vi "Read.vi"(7 "I2C Channel (0)":u8, 8 "Error In":errorcluster, 10 "TCN75A I2C Address":T7, 11 "LINX Resource":T1) -> (0 "Error Out":errorcluster, 1 "Temp F":dbl, 2 "Temp C":dbl, 3 "LINX Resource":T1)   [LabVIEW 2011, in "LVH-LINX.lvlib" / "TCN75A.lvlib"]
doc: "Read temperature from the TCN75A."
uses:
  TCN75A.lvlib
  Private/Type Defs/LINX Ref.ctl
  Private/Type Defs/Platform.ctl
  Private/Type Defs/Interface.ctl
  Private/Device/Type Defs/LINX Device Config.ctl
  Private/Device/Type Defs/TCP Config.ctl
  Private/Device/Type Defs/Channels.ctl
  I2C Address.ctl
  LVH-LINX.lvlib
  Private/Device/Device.lvlib
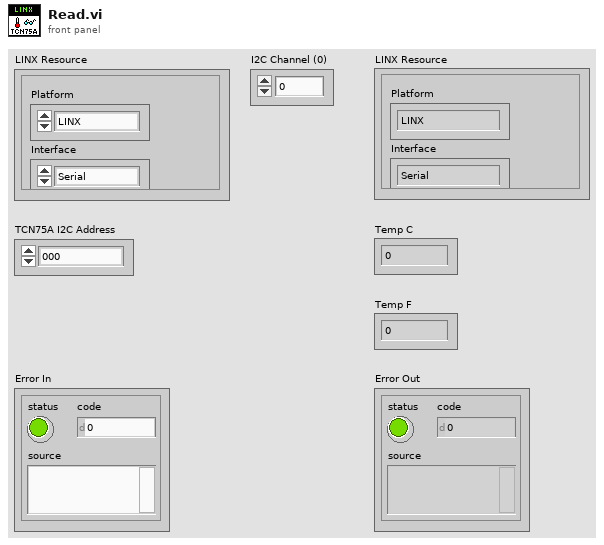
[diagram p1: front panel]
types:
  T1 = typedef "LVH-LINX.lvlib/LINX Ref.ctl" = cluster{"Platform":T2, "Interface":T3, "LINX Device Config":T4}
  T2 = typedef "LVH-LINX.lvlib/Platform.ctl" = enum16{"LINX", "myRIO"}
  T3 = typedef "LVH-LINX.lvlib/Interface.ctl" = enum16{"Serial", "TCP"}
  T4 = typedef "LVH-LINX.lvlib/Device.lvlib/LINX Device Config.ctl" = cluster{"Interface":T3, "COM Port":refnum<visa-resource-name>, "TCP Configuration":T5, "Device Family":u8, "Device ID":u8, "Device Name":string, "TCP Ref":refnum<k5>, "Channels":T6}
  T5 = typedef "LVH-LINX.lvlib/Device.lvlib/TCP Config.ctl" = cluster{"IP Address":string, "Port":u16}
  T6 = typedef "LVH-LINX.lvlib/Channels.ctl" = cluster{"DI Channels":u8[], "DO Channels":u8[], "AI":u8[], "AO":u8[], "PWM":u8[], "QE":u8[], "UART":u8[], "I2C 2":u8[], "SPI":u8[], "CAN":u8[], "AI Ref (V)":dbl, "AO Resolution (Bits)":u8, "AO Ref (V)":dbl}
  T7 = typedef "LVH-LINX.lvlib/TCN75A.lvlib/I2C Address.ctl" = enum8{"000", "001", "010", "011", "100", "101", "110", "111"}
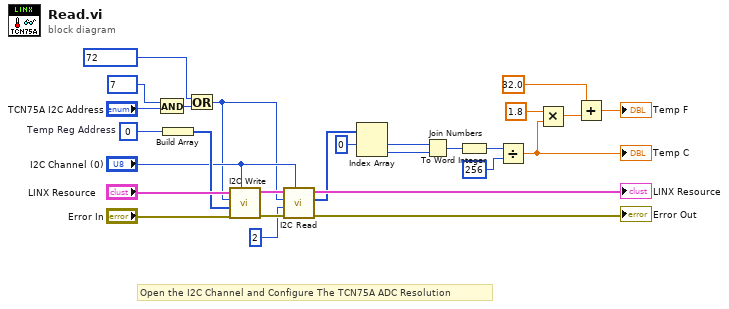
[diagram p0: block diagram]
diagram:
  w25 = u8 0  # Temp Reg Address
  # "Open the I2C Channel and Configure The TCN75A ADC Resolution"
  n1 = And(x=u8 7, y="TCN75A I2C Address") -> (x .and. y?=w15:u8)
  n2 = Build Array(w25) -> (w24:u8[])
  n3 = Or(x=u8 72, y=w15) -> (x .or. y?=w13:u8)
  n4 = call "I2C Write.vi"("I2C Channel"="I2C Channel (0)", "Error In"="Error In", "Data"=w24, "I2C Slave Address (0)"=w13, "LINX Resource"="LINX Resource") -> ("Error Out"=w22:errorcluster, "LINX Resource"=w23:T1)  [unwired: 5 in]
  n5 = call "I2C Read.vi"("I2C Channel"="I2C Channel (0)", "Error In"=w22, "Bytes To Read"=u8 2, "I2C Slave Address (0)"=w13, "LINX Resource"=w23) -> ("Error Out"=→"Error Out":errorcluster, "Data"=w12:u8[], "LINX Resource"=→"LINX Resource":T1)  [unwired: 4 in]
  n6 = Index Array(array=w12, index #1=0 ("index")) -> (element #1=w10:u8, element #2=w9:u8)  [unwired: 1 in]
  n7 = Join Numbers(hi=w10, lo=w9) -> ((hi.lo)=w8:u16)
  n8 = To Word Integer(number=w8) -> (16bit integer=w7:i16)
  n9 = Divide(x=w7, y=i16 256) -> (x/y=w5:dbl)
  "Temp C" <- w5
  n10 = Multiply(x=1.8, y=w5) -> (x*y=w3:dbl)
  n11 = Add(x=32.0, y=w3) -> (x+y=→"Temp F":dbl)
